vi "DRWM模块_两列DSF.vi"(1 "通量名称":string[](array[string]), 2 "因子说明":string, 3 "P2名称":string[](array[string]), 5 "SSF因子":cluster{"x":dbl, "y":dbl}[][](array[cluster]), 7 "因子棒名":string[](array[string]), 9 "时间步长":sgl, 11 "通量in":dbl[][](array[numeric]), 12 "执行:调用时显示前面板":bool, 14 "P2信号":dbl[][](array[numeric])) -> (0 "通量out":dbl[][](array[numeric]), 4 "上下段通量索引":u16[](array[numeric]), 6 "动态因子棒选择":u16, 8 "P2信号out":dbl[][](array[numeric]), 10 "DRWM开":bool, 13 "棒限":dbl[](array[numeric]), 15 "动态棒位":dbl[](array[numeric]))   [LabVIEW 2020]
uses:
  <vilib>/Analysis/baseanly.llb/Mean (DBL).vi
  <vilib>/Analysis/NI_AALBase.lvlib
panel:
  in  "核星DSF":bool
  in  "修正因子选择":u16(ring)
  out "修正因子文件说明":string
  in  "底部棒位(步)":dbl=5.0
  in  "触发准备":bool
  out "触发量稳定值":dbl
  in  "通量触发选择":u16(ring)=2 items=["电流1a", "电流2a"]
  out "触发量散度%":dbl
  in  "触发量容限%":dbl=10.0
  in  "通量暂存":dbl[](array[numeric])
  in  "棒位暂存":dbl[](array[numeric])
  in  "触发方式":u16(ring)=2 items=["手动触发启动", "通量触发启动", "棒位触发启动", "实时棒位无需触发"]
  in  "顶部棒位(步)":dbl=225.0
  out "面板开":bool
  in  "棒速(步/分钟)":dbl=72.0
  out "DRWM控制棒":dbl(slide) min=0.0 max=225.0 scale=0.0..225.0
  in  "DRWM启动":bool
  in  "上部探测器选择":u16(ring) items=["电流1a", "电流2a"]
  in  "下部探测器选择":u16(ring)=1 items=["电流1a", "电流2a"]
  in  "控制棒选择":i32(ring) items=["D棒位", "C棒位"]
  # "NPIC DSF"
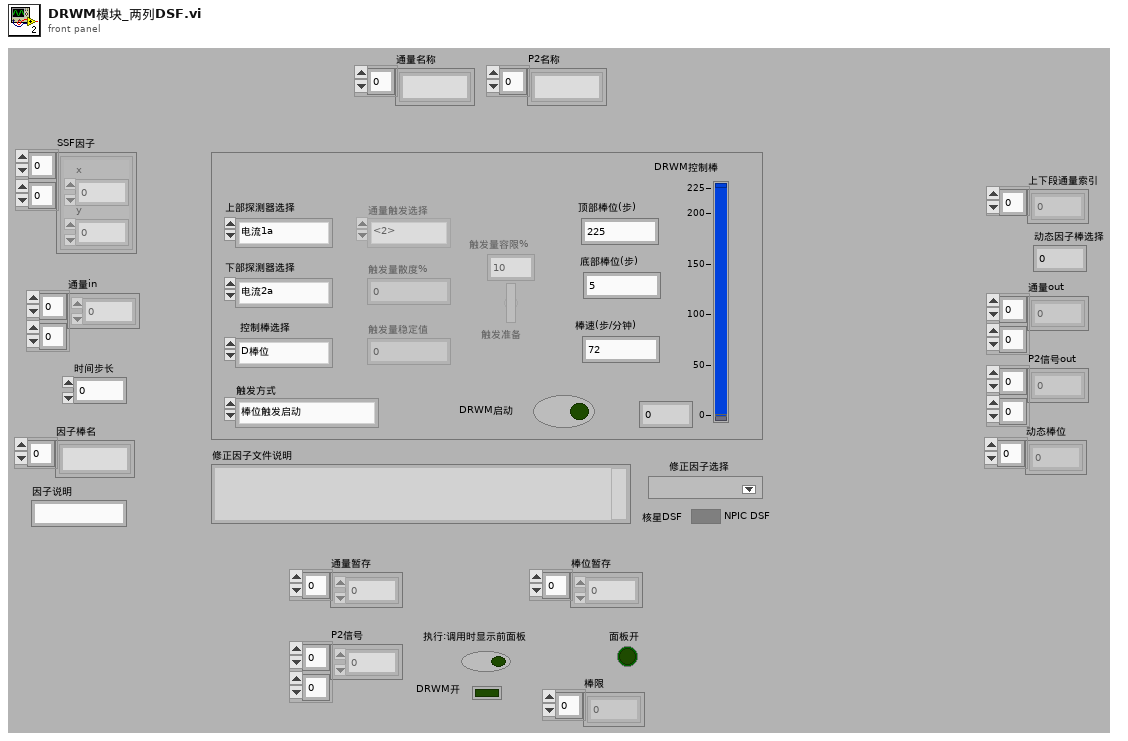
[diagram p1: front panel]
types:
  T1 = enum8{"Enabled", "Disabled", "Disabled and Grayed Out"}
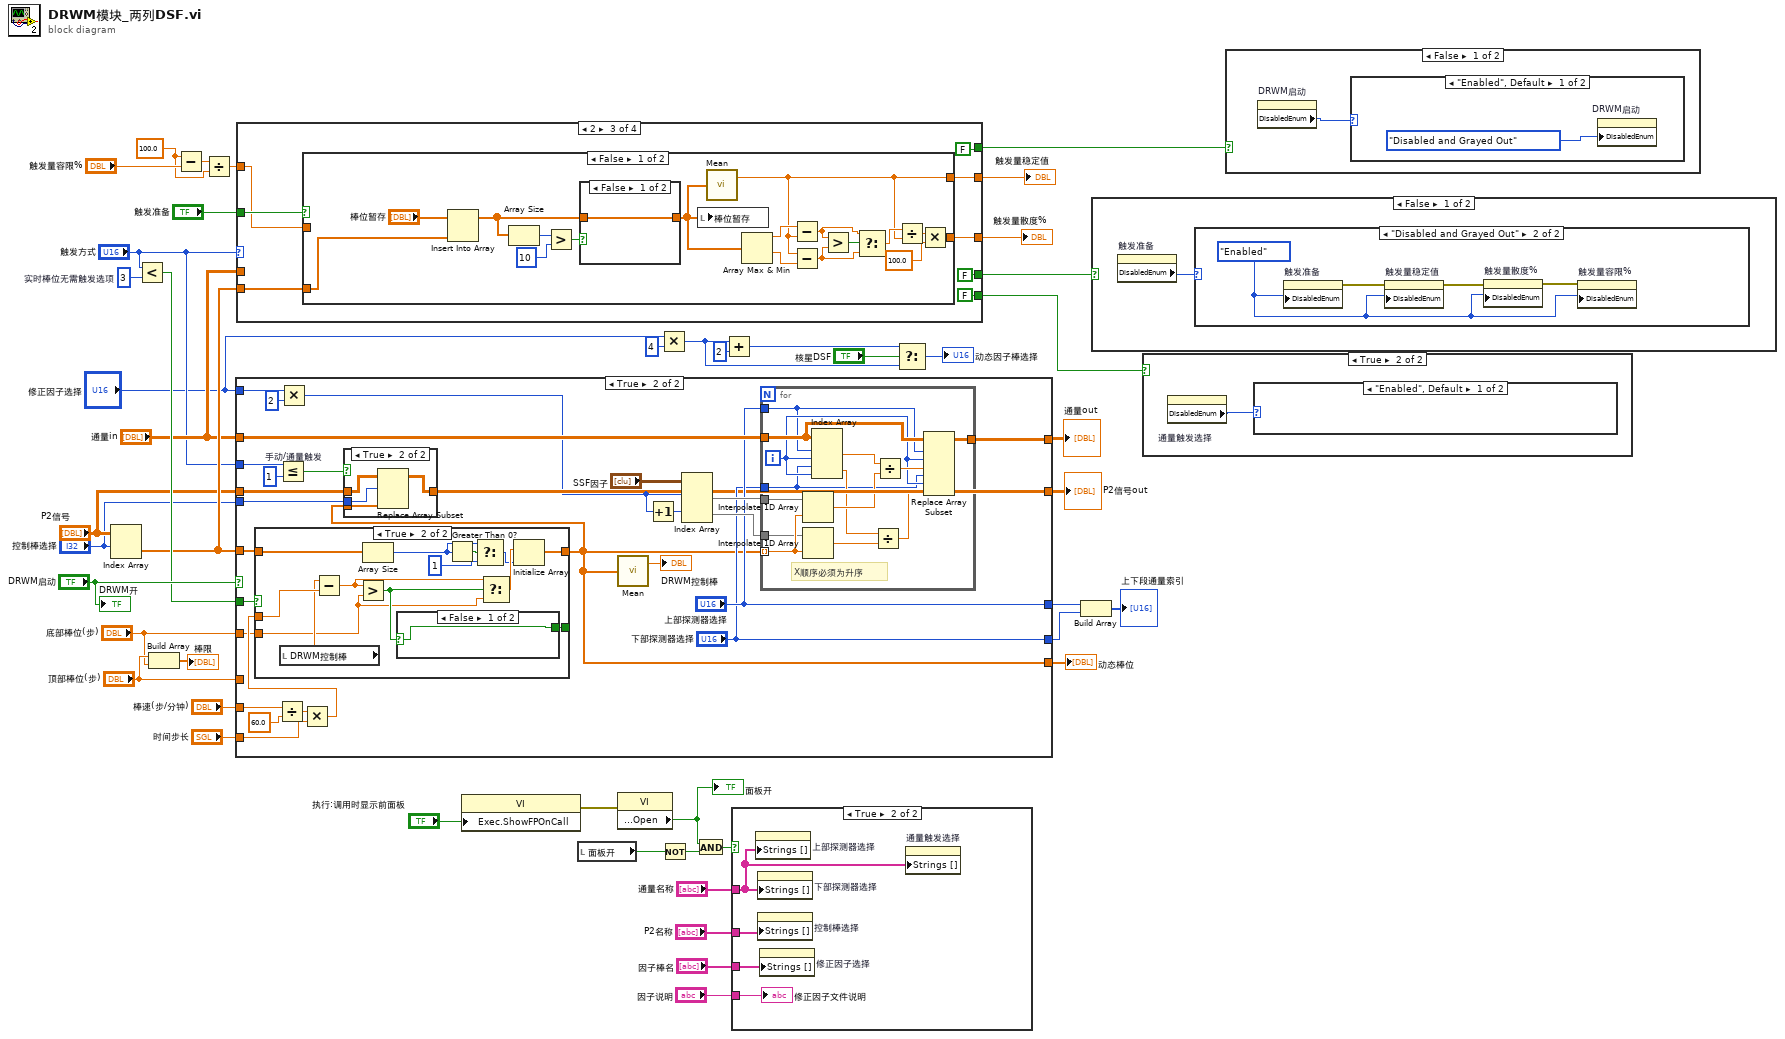
[diagram p0: block diagram]
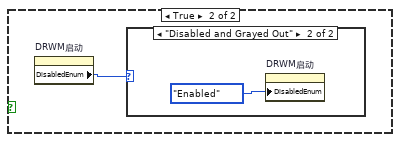
[diagram p3: hidden frame]
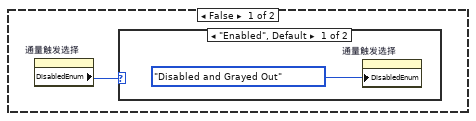
[diagram p5: hidden frame]
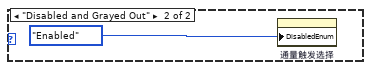
[diagram p7: hidden frame]
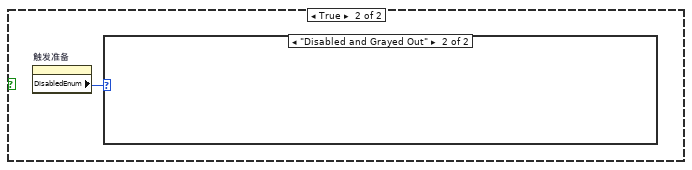
[diagram p9: hidden frame]
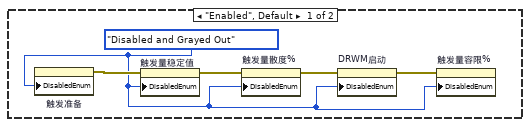
[diagram p10: hidden frame]
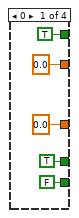
[diagram p11: hidden frame]
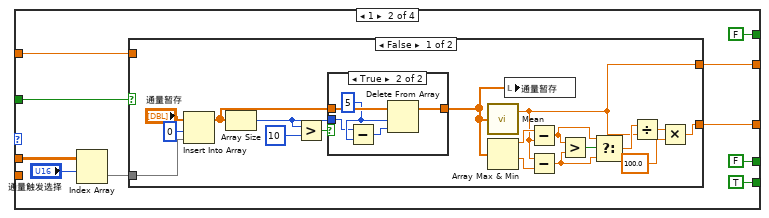
[diagram p12: hidden frame]
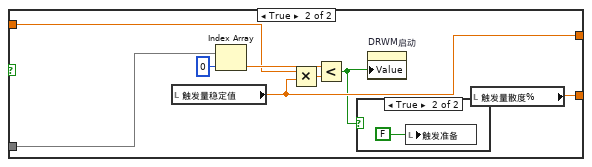
[diagram p14: hidden frame]
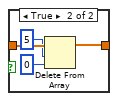
[diagram p16: hidden frame]
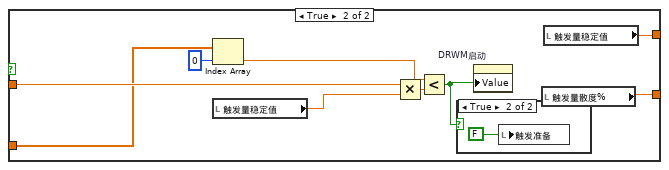
[diagram p17: hidden frame]
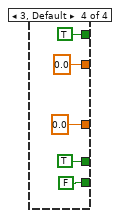
[diagram p19: hidden frame]
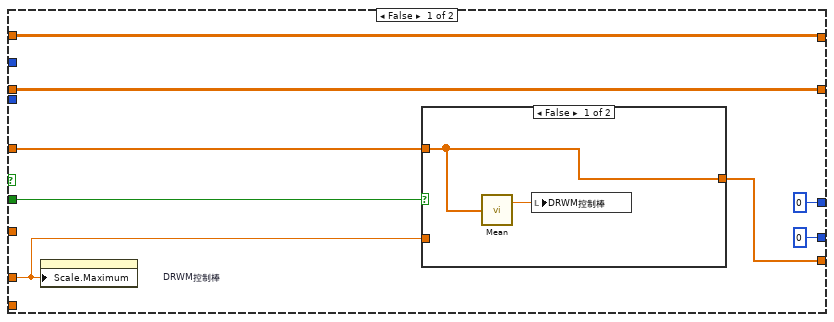
[diagram p20: hidden frame]
diagram:
  w30 = 100.0 ("x")
  w34 = u16 3  # 实时棒位无需触发选项
  n1 = Index Array(array="P2信号", index (row)="控制棒选择") -> (element=w29:dbl[])  [unwired: 1 in]
  n2 = Less?(x="触发方式", y=w34) -> (x < y?=w35:bool)
  n3 = Build Array("顶部棒位(步)", "底部棒位(步)") -> (→"棒限":dbl[])
  n4 = Subtract(x=w30, y="触发量容限%") -> (x-y=w31:dbl)
  n5 = Divide(x=w31, y=w30) -> (x/y=w28:dbl)
  n6 = case shown="True" "DRWM启动" {
    tunnel: "通量in" -> [w54 w90]
    tunnel: [w54 w89] -> w40
    tunnel: "棒速(步/分钟)" -> [_ w84]
    tunnel: "时间步长" -> [_ w78]
    tunnel: "顶部棒位(步)" -> [w48 _]
    tunnel: w35 -> [w49 w82]
    tunnel: w29 -> [w50 w81]
    tunnel: [u16 0 ("上部探测器选择") "上部探测器选择"] -> w10
    tunnel: [u16 0 ("下部探测器选择") "下部探测器选择"] -> w9
    tunnel: [w51 w70] -> w25
    tunnel: "P2信号" -> [w47 w72]
    tunnel: [w47 w71] -> w18
    tunnel: "触发方式" -> [_ w75]
    tunnel: "控制棒选择" -> [_ w69]
    tunnel: "底部棒位(步)" -> [_ w68]
    tunnel: "修正因子选择" -> [_ w67]
    frame False {
      n7 = property on="DRWM控制棒" class="Slide (strict)"("Scale.Maximum"=w48) -> ()  [unwired: 2 in, 2 out]
      n8 = case shown="False" w49 {
        tunnel: [w55 w60] -> w51
        tunnel: w50 -> [w55 w59]
        tunnel: w48 -> [_ w57]
        frame False {
          n9 = call-poly <vilib>:"Mean.vi"("X"=w55) -> ("mean"=w56:dbl)  [unwired: 1 out]
          n10 = local write "DRWM控制棒"(w56) -> ()
        }
        frame True {
          n11 = local write "DRWM控制棒"(w57) -> ()
          n12 = Array Size(array=w59) -> (size(s)=w58:i32)
          n13 = Greater Than 0?(x=w58) -> (x > 0?=w63:bool)
          n14 = Select(t=w58, s=w63, f=1) -> (s? t:f=w62:i32)
          n15 = Initialize Array(w57, w62) -> (w60:dbl[])
        }
      }
    }
    frame True {
      w74 = u16 1  # 手动/通量触发
      n16 = Divide(x=w84, y=60.0) -> (x/y=w77:dbl)
      n17 = Less Or Equal?(x=w75, y=w74) -> (x <= y?=w73:bool)
      n18 = Multiply(x=w67, y=u16 2) -> (x*y=w64:u16)
      n19 = Multiply(x=w77, y=w78) -> (x*y=w76:dbl)
      n20 = case shown="True" w82 {
        tunnel: w81 -> [w99 w112]
        tunnel: [w99 w111] -> w70
        tunnel: w76 -> [_ w110]
        tunnel: w68 -> [w97 w100]
        tunnel: [w96 w102] -> _
        frame False {
          n21 = call-poly <vilib>:"Mean.vi"("X"=w99) -> ("mean"=w98:dbl)  [unwired: 1 out]
          n22 = Greater?(x=w98, y=w97) -> (0:w96:bool)
        }
        frame True {
          n23 = local read "DRWM控制棒"() -> (w101:dbl)
          n24 = Subtract(x=w101, y=w110) -> (x-y=w103:dbl)
          n25 = Greater?(x=w103, y=w100) -> (0:w104:bool)
          n26 = Array Size(array=w112) -> (size(s)=w106:i32)
          n27 = case shown="False" w104 {
            selector: w104 -> [w113 w114]
            tunnel: [w113 w114] -> w102
            frame False {
            }
            frame True {
            }
          }
          n28 = Greater Than 0?(x=w106) -> (x > 0?=w108:bool)
          n29 = Select(t=w106, s=w108, f=1) -> (s? t:f=w107:i32)
          n30 = Select(t=w103, s=w104, f=w100) -> (s? t:f=w109:dbl)
          n31 = Initialize Array(w109, w107) -> (w111:dbl[])
        }
      }
      n32 = case shown="True" w73 {
        tunnel: w72 -> [w91 w95]
        tunnel: [w91 w94] -> w71
        tunnel: w70 -> [_ w93]
        tunnel: w69 -> [_ w92]
        frame False {
        }
        frame True {
          n33 = Replace Array Subset(array=w95, new element=w93, index (row)=w92) -> (w94:dbl[][])  [unwired: 1 in]
        }
      }
      n34 = call-poly <vilib>:"Mean.vi"("X"=w70) -> ("mean"=→"DRWM控制棒":dbl)  [unwired: 1 out]
      n35 = Increment(x=w64) -> (x+1=w65:u16)
      n36 = Index Array(array="SSF因子", index (row) #1=w64, index (row) #2=w65) -> (element #1=w87:cluster{"x":dbl, "y":dbl}[], element #2=w86:cluster{"x":dbl, "y":dbl}[])  [unwired: 2 in]
      n37 = for {
        tunnel: w70 -> [w122] mode=indexing
        tunnel: w87 -> [w128]
        tunnel: w90 -> [w127]
        tunnel: [w126] -> w89
        tunnel: w86 -> [w117]
        tunnel: "上部探测器选择" -> [w116]
        tunnel: "下部探测器选择" -> [w115]
        i -> [w118]
        # "X顺序必须为升序"
        n38 = Interpolate 1D Array(1:w122, 2:w128) -> (0:w123:dbl)
        n39 = Interpolate 1D Array(1:w122, 2:w117) -> (0:w121:dbl)
        n40 = Index Array(array=w127, index (row) #1=w116, index (col) #1=w118, index (row) #2=w115, index (col) #2=w118) -> (element #1=w125:dbl, element #2=w120:dbl)
        n41 = Divide(x=w120, y=w121) -> (x/y=w119:dbl)
        n42 = Divide(x=w125, y=w123) -> (x/y=w124:dbl)
        n43 = Replace Array Subset(array=w127, new element #1=w124, index (row) #1=w116, index (col) #1=w118, new element #2=w119, index (row) #2=w115, index (col) #2=w118) -> (w126:dbl[][])
      }
    }
  }
  "通量out" <- w40
  "动态棒位" <- w25
  "P2信号out" <- w18
  n44 = case shown="2" "触发方式" {
    tunnel: w29 -> [_ _ w184 _]
    tunnel: w28 -> [_ w137 w181 _]
    tunnel: "通量in" -> [_ w139 _ _]
    tunnel: [0.0 ("触发量散度%") w143 w183 0.0] -> w26
    tunnel: [0.0 ("mean") w142 w180 0.0 ("触发量稳定值")] -> w24
    tunnel: "触发准备" -> [_ w138 w182 _]
    tunnel: [TRUE FALSE FALSE TRUE] -> w22
    tunnel: [FALSE TRUE FALSE FALSE] -> w21
    tunnel: [TRUE FALSE FALSE TRUE] -> w20
    frame 0 {
    }
    frame 1 {
      n45 = Index Array(array=w139, index (row)="通量触发选择") -> (element=w140:dbl[])  [unwired: 1 in]
      n46 = case shown="False" w138 {
        tunnel: [w146 w175] -> w143
        tunnel: [w145 w171] -> w142
        tunnel: w140 -> [w144 w170]
        tunnel: w137 -> [_ w168]
        frame False {
          n47 = Insert Into Array(array="通量暂存", index=0 ("索引"), new element=w144) -> (w158:dbl[])
          n48 = Array Size(array=w158) -> (size(s)=w156:i32)
          n49 = Greater?(x=w156, y=10) -> (0:w161:bool)
          n50 = case shown="True" w161 {
            tunnel: w158 -> [w162 w166]
            tunnel: [w162 w167] -> w157
            tunnel: w156 -> [_ w164]
            frame False {
            }
            frame True {
              w165 = 5 ("长度")
              n51 = Subtract(x=w164, y=w165) -> (x-y=w163:i32)
              n52 = Delete From Array(array=w166, length=w165, index=w163) -> (array with subset deleted=w167:dbl[])  [unwired: 1 out]
            }
          }
          n53 = call-poly <vilib>:"Mean.vi"("X"=w157) -> ("mean"=w145:dbl)  [unwired: 1 out]
          n54 = Array Max & Min(array=w157) -> (max value=w154:dbl, min value=w153:dbl)  [unwired: 2 out]
          n55 = local write "通量暂存"(w157) -> ()
          n56 = Subtract(x=w154, y=w145) -> (x-y=w151:dbl)
          n57 = Subtract(x=w145, y=w153) -> (x-y=w150:dbl)
          n58 = Greater?(x=w151, y=w150) -> (0:w152:bool)
          n59 = Select(t=w151, s=w152, f=w150) -> (s? t:f=w149:dbl)
          n60 = Divide(x=w149, y=w145) -> (x/y=w148:dbl)
          n61 = Multiply(x=w148, y=100.0) -> (x*y=w146:dbl)
        }
        frame True {
          n62 = local read "触发量稳定值"() -> (w171:dbl)
          n63 = Index Array(array=w170, index=0 ("索引")) -> (element=w173:dbl)
          n64 = Multiply(x=w168, y=w171) -> (x*y=w172:dbl)
          n65 = Less?(x=w173, y=w172) -> (x < y?=w169:bool)
          n66 = case shown="True" w169 {
            frame False {
            }
            frame True {
              n67 = local write "触发准备"(FALSE ("触发准备")) -> ()
            }
          }
          n68 = property on="DRWM启动" class="Bool (strict)"("Value"=w169) -> ()  [unwired: 2 in, 2 out]
          n69 = local read "触发量散度%"() -> (w175:dbl)
        }
      }
    }
    frame 2 {
      n70 = case shown="False" w182 {
        tunnel: w184 -> [w196 w210]
        tunnel: [w186 w214] -> w183
        tunnel: w181 -> [_ w212]
        tunnel: [w185 w207] -> w180
        frame False {
          n71 = Insert Into Array(array="棒位暂存", new element=w196) -> (w200:dbl[])  [unwired: 1 in]
          n72 = Array Size(array=w200) -> (size(s)=w198:i32)
          n73 = Greater?(x=w198, y=10) -> (0:w201:bool)
          n74 = case shown="False" w201 {
            tunnel: w200 -> [w202 w205]
            tunnel: [w202 w206] -> w192
            frame False {
            }
            frame True {
              n75 = Delete From Array(array=w205, length=5 ("长度"), index=0 ("索引")) -> (array with subset deleted=w206:dbl[])  [unwired: 1 out]
            }
          }
          n76 = local write "棒位暂存"(w192) -> ()
          n77 = call-poly <vilib>:"Mean.vi"("X"=w192) -> ("mean"=w185:dbl)  [unwired: 1 out]
          n78 = Array Max & Min(array=w192) -> (max value=w191:dbl, min value=w195:dbl)  [unwired: 2 out]
          n79 = Subtract(x=w191, y=w185) -> (x-y=w190:dbl)
          n80 = Subtract(x=w185, y=w195) -> (x-y=w193:dbl)
          n81 = Greater?(x=w190, y=w193) -> (0:w194:bool)
          n82 = Select(t=w190, s=w194, f=w193) -> (s? t:f=w187:dbl)
          n83 = Divide(x=w187, y=w185) -> (x/y=w189:dbl)
          n84 = Multiply(x=w189, y=100.0) -> (x*y=w186:dbl)
        }
        frame True {
          n85 = Index Array(array=w210, index=0 ("索引")) -> (element=w209:dbl)
          n86 = local read "触发量稳定值"() -> (w213:dbl)
          n87 = Multiply(x=w212, y=w213) -> (x*y=w215:dbl)
          n88 = Less?(x=w209, y=w215) -> (x < y?=w208:bool)
          n89 = case shown="True" w208 {
            frame False {
            }
            frame True {
              n90 = local write "触发准备"(FALSE ("触发准备")) -> ()
            }
          }
          n91 = property on="DRWM启动" class="Bool (strict)"("Value"=w208) -> ()  [unwired: 2 in, 2 out]
          n92 = local read "触发量散度%"() -> (w214:dbl)
          n93 = local read "触发量稳定值"() -> (w207:dbl)
        }
      }
    }
    frame 3, Default {
    }
  }
  "触发量散度%" <- w26
  "触发量稳定值" <- w24
  n94 = property class="VI"("Exec.ShowFPOnCall"="执行:调用时显示前面板") -> (error out=w45:errorcluster)  [unwired: 2 in, 1 out]
  n95 = local read "面板开"() -> (w44:bool)
  n96 = property class="VI"(error in=w45) -> ("Front Panel.Open"=w42:bool)  [unwired: 1 in, 2 out]
  "面板开" <- w42
  n97 = Multiply(x="修正因子选择", y=u16 4) -> (x*y=w2:u16)
  n98 = Not(x=w44) -> (.not. x?=w43:bool)
  n99 = And(x=w42, y=w43) -> (x .and. y?=w41:bool)
  n100 = Add(x=w2, y=u16 2) -> (x+y=w1:u16)
  n101 = case shown="True" w41 {
    tunnel: "P2名称" -> [_ w225]
    tunnel: "通量名称" -> [_ w224]
    tunnel: "因子棒名" -> [_ w222]
    tunnel: "因子说明" -> [_ w223]
    frame False {
    }
    frame True {
      n102 = property on="上部探测器选择" class="Ring (strict)"("Strings []"=w224) -> ()  [unwired: 2 in, 2 out]
      n103 = property on="下部探测器选择" class="Ring (strict)"("Strings []"=w224) -> ()  [unwired: 2 in, 2 out]
      n104 = property on="控制棒选择" class="Ring (strict)"("Strings []"=w225) -> ()  [unwired: 2 in, 2 out]
      n105 = property on="修正因子选择" class="Ring (strict)"("Strings []"=w222) -> ()  [unwired: 2 in, 2 out]
      n106 = property on="通量触发选择" class="Ring (strict)"("Strings []"=w224) -> ()  [unwired: 2 in, 2 out]
      "修正因子文件说明" <- w223
    }
  }
  n107 = Select(t=w1, s="核星DSF", f=w2) -> (s? t:f=→"动态因子棒选择":u16)
  n108 = Build Array(w10, w9) -> (→"上下段通量索引":u16[])
  n109 = case shown="False" w22 {
    frame False {
      n110 = property on="触发准备" class="Bool (strict)"() -> ("DisabledEnum"=w226:T1)  [unwired: 2 in, 2 out]
      n111 = case shown="\"Disabled and Grayed Out\"" w226 {
        frame "Enabled", Default {
        }
        frame "Disabled and Grayed Out" {
          w228 = T1."Enabled" ("禁用")
          n112 = property on="触发准备" class="Bool (strict)"("DisabledEnum"=w228) -> (error out=w230:errorcluster)  [unwired: 2 in, 1 out]
          n113 = property on="触发量稳定值" class="DigNum (strict)"(error in=w230, "DisabledEnum"=w228) -> (error out=w229:errorcluster)  [unwired: 1 in, 1 out]
          n114 = property on="触发量散度%" class="DigNum (strict)"(error in=w229, "DisabledEnum"=w228) -> (error out=w227:errorcluster)  [unwired: 1 in, 1 out]
          n115 = property on="触发量容限%" class="DigNum (strict)"(error in=w227, "DisabledEnum"=w228) -> ()  [unwired: 1 in, 2 out]
        }
      }
    }
    frame True {
      n116 = property on="触发准备" class="Bool (strict)"() -> ("DisabledEnum"=w231:T1)  [unwired: 2 in, 2 out]
      n117 = case shown="\"Disabled and Grayed Out\"" w231 {
        frame "Enabled", Default {
          w232 = T1."Disabled and Grayed Out" ("禁用")
          n118 = property on="触发准备" class="Bool (strict)"("DisabledEnum"=w232) -> (error out=w235:errorcluster)  [unwired: 2 in, 1 out]
          n119 = property on="触发量稳定值" class="DigNum (strict)"(error in=w235, "DisabledEnum"=w232) -> (error out=w236:errorcluster)  [unwired: 1 in, 1 out]
          n120 = property on="触发量散度%" class="DigNum (strict)"(error in=w236, "DisabledEnum"=w232) -> (error out=w234:errorcluster)  [unwired: 1 in, 1 out]
          n121 = property on="DRWM启动" class="Bool (strict)"(error in=w234, "DisabledEnum"=w232) -> (error out=w233:errorcluster)  [unwired: 1 in, 1 out]
          n122 = property on="触发量容限%" class="DigNum (strict)"(error in=w233, "DisabledEnum"=w232) -> ()  [unwired: 1 in, 2 out]
        }
        frame "Disabled and Grayed Out" {
        }
      }
    }
  }
  n123 = case shown="True" w21 {
    frame False {
      n124 = property on="通量触发选择" class="Ring (strict)"() -> ("DisabledEnum"=w237:T1)  [unwired: 2 in, 2 out]
      n125 = case shown="\"Enabled\", Default" w237 {
        frame "Enabled", Default {
          n126 = property on="通量触发选择" class="Ring (strict)"("DisabledEnum"=T1."Disabled and Grayed Out" ("禁用")) -> ()  [unwired: 2 in, 2 out]
        }
        frame "Disabled and Grayed Out" {
        }
      }
    }
    frame True {
      n127 = property on="通量触发选择" class="Ring (strict)"() -> ("DisabledEnum"=w239:T1)  [unwired: 2 in, 2 out]
      n128 = case shown="\"Enabled\", Default" w239 {
        frame "Enabled", Default {
        }
        frame "Disabled and Grayed Out" {
          n129 = property on="通量触发选择" class="Ring (strict)"("DisabledEnum"=T1."Enabled" ("禁用")) -> ()  [unwired: 2 in, 2 out]
        }
      }
    }
  }
  n130 = case shown="False" w20 {
    frame False {
      n131 = property on="DRWM启动" class="Bool (strict)"() -> ("DisabledEnum"=w241:T1)  [unwired: 2 in, 2 out]
      n132 = case shown="\"Enabled\", Default" w241 {
        frame "Enabled", Default {
          n133 = property on="DRWM启动" class="Bool (strict)"("DisabledEnum"=T1."Disabled and Grayed Out" ("禁用")) -> ()  [unwired: 2 in, 2 out]
        }
        frame "Disabled and Grayed Out" {
        }
      }
    }
    frame True {
      n134 = property on="DRWM启动" class="Bool (strict)"() -> ("DisabledEnum"=w243:T1)  [unwired: 2 in, 2 out]
      n135 = case shown="\"Disabled and Grayed Out\"" w243 {
        frame "Enabled", Default {
        }
        frame "Disabled and Grayed Out" {
          n136 = property on="DRWM启动" class="Bool (strict)"("DisabledEnum"=T1."Enabled" ("禁用")) -> ()  [unwired: 2 in, 2 out]
        }
      }
    }
  }
  "DRWM开" <- "DRWM启动"
